vi "tearDown.vi"(8 "error in (no error)":errorcluster, 11 "reference in":refnum<class "Verify IMemento.lvclass">) -> (0 "error out":errorcluster, 3 "reference out":refnum<class "Verify IMemento.lvclass">)   [LabVIEW 2009, in "Verify IMemento.lvclass"]
doc: "tearDown runs after the test method has completed. Use this method to clean up any operations or references that were opened by setUp or the test method. Unit tests should be independent of other unit tests so this VI should ensure that the next test can run in a 'clean' test environment."
uses:
  Verify IMemento.lvclass
  Verify IMemento.lvclass/Verify IMemento.ctl
  Numeric Test Object/Numeric Test Object.lvclass
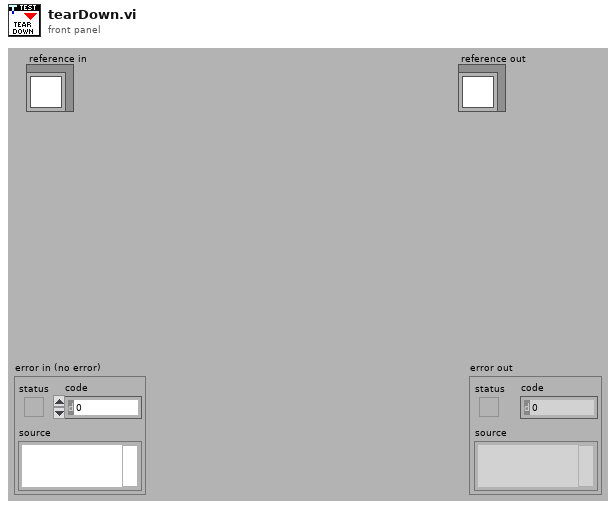
[diagram p1: front panel]
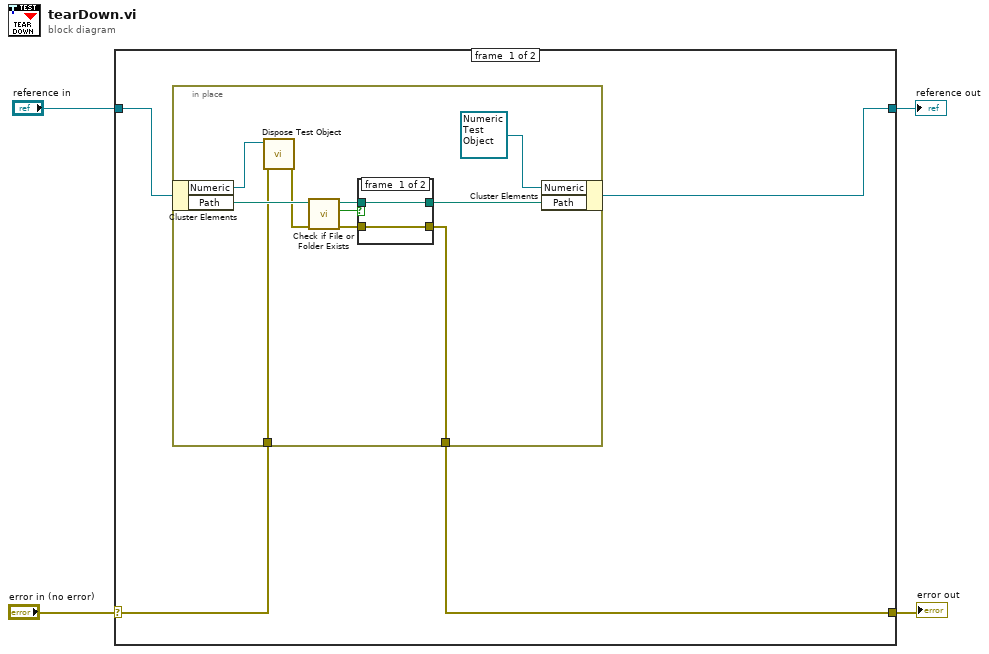
[diagram p0: block diagram]
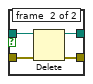
[diagram p2: hidden frame]
diagram:
  n1 = case shown="No Error" "error in (no error)" {
    selector: "error in (no error)" -> [w6 w26]
    tunnel: [w5 w26] -> w3
    tunnel: [w7 w25] -> w1
    tunnel: "reference in" -> [w8 w25]
    frame #0 {
      n2 = in-place {
        in-place-border: w6 -> [w15]
        in-place-border: [w10] -> w5
        n3 = in-place-cluster #1(w8) -> ("Numeric"=w18:refnum<class "Numeric Test Object.lvclass">, "Path"=w16:path)
        n4 = call "Dispose Test Object.vi"("error in (no error)"=w15, "Numeric"=w18) -> ("error out"=w14:errorcluster)  [unwired: 9 in]
        n5 = call <vilib>:"Check if File or Folder Exists.vi"("error in (no error)"=w14, "path"=w16) -> ("error out"=w11:errorcluster, "file or folder exists?"=w13:bool, "dup path"=w12:path)  [unwired: 7 in]
        n6 = case shown="True" w13 {
          tunnel: w12 -> [w19 w24]
          tunnel: w11 -> [w20 w23]
          tunnel: [w20 w22] -> w10
          tunnel: [w19 w21] -> w9
          frame #0 {
          }
          frame #1 {
            n7 = Delete(path (use dialog)=w24, error in=w23) -> (deleted path=w21:path, error out=w22:errorcluster)  [unwired: 3 in, 1 out]
          }
        }
        n8 = in-place-cluster #1("Numeric"=refnum<class "Numeric Test Object.lvclass"> refnum, "Path"=w9) -> (w7:refnum<class "Verify IMemento.lvclass">)
      }
    }
    frame #1 {
    }
  }
  "error out" <- w3
  "reference out" <- w1
